vi "ImageProcessing_Main.vi"() -> ()   [LabVIEW 2020]
uses:
  #typedef_ImPro_InputData.ctl
  #typedef_states.ctl
  #typedef_ImagePath.ctl
panel:
  in  "Sharp":bool
  in  "Blur":bool
  in  "Gauss":bool
  in  "Binaryzacja":bool
  in  "stop":bool
  in  "Load Picture":bool
  in  "Path":path
  out "Output Image":picture
  out "Input Image":picture
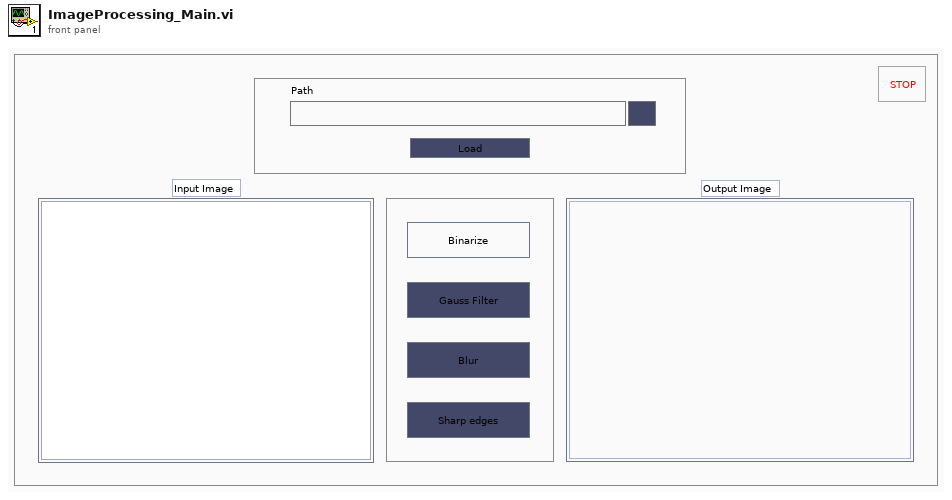
[diagram p1: front panel]
types:
  T1 = typedef "#typedef_ImagePath.ctl" = cluster{"Image path":path}
  T2 = typedef "#typedef_ImPro_InputData.ctl" = cluster{"Command":T3, "Data":variant}
  T3 = typedef "#typedef_states.ctl" = enum16{"Rozmycie", "Wyostrzenie", "Gauss", "Binaryzacja", "Load Picture", "Exit"}
  T4 = typedef "imagedata.ctl" = cluster{"image type":i32, "image depth":i32, "image":u8[], "mask":u8[], "colors":u32[], "Rectangle":cluster{"left":i16, "top":i16, "right":i16, "bottom":i16}}
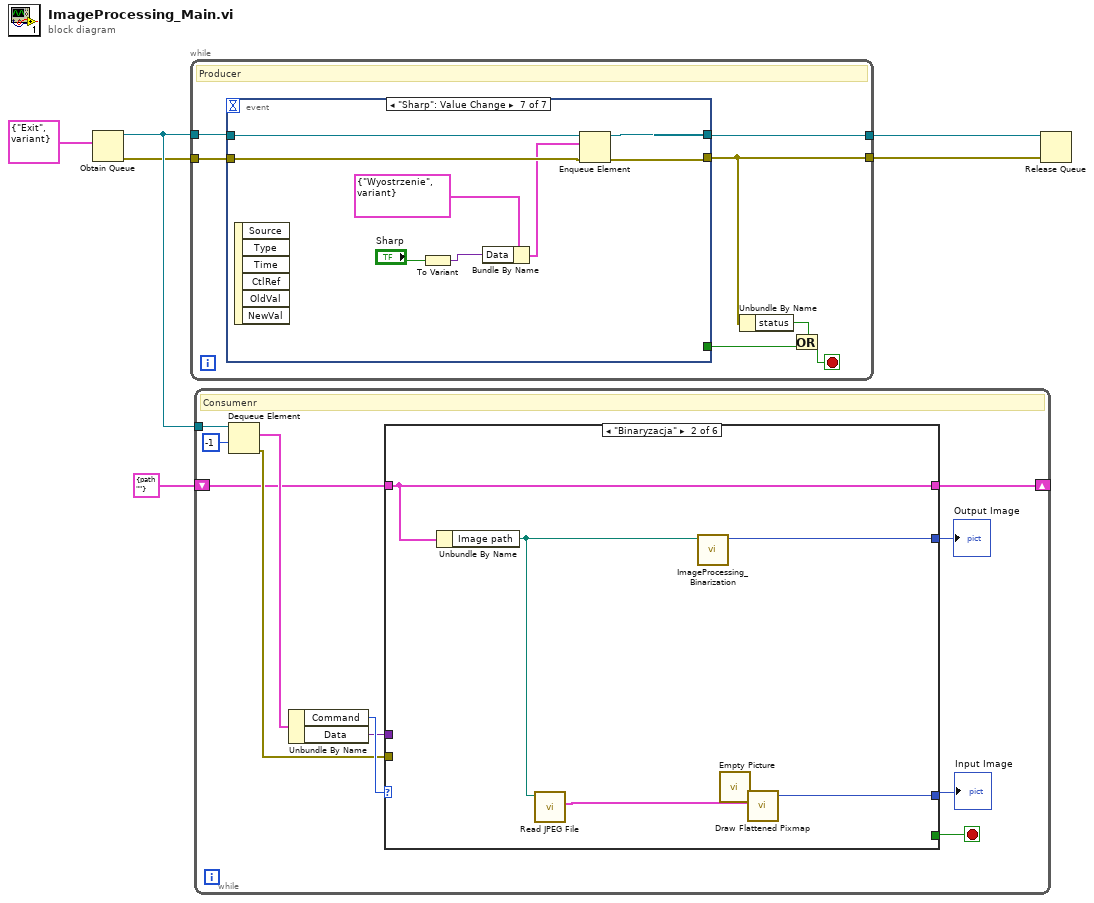
[diagram p0: block diagram]
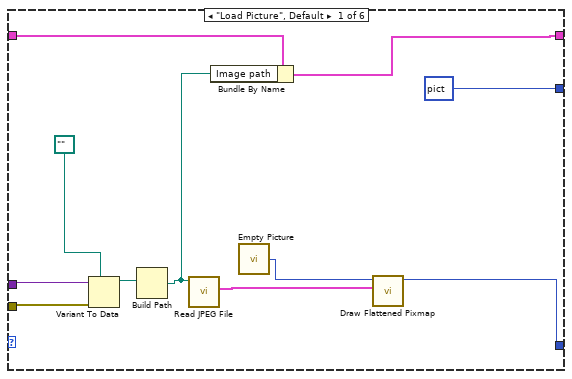
[diagram p2: hidden frame]
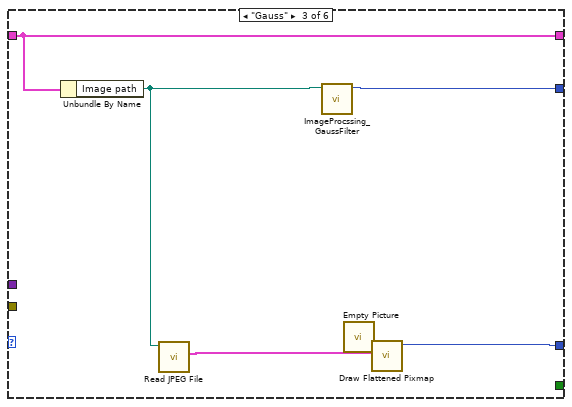
[diagram p3: hidden frame]
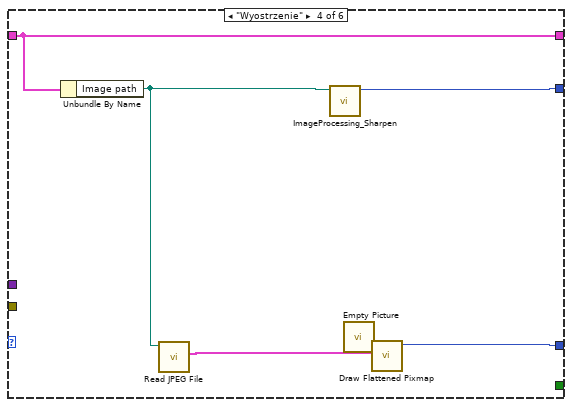
[diagram p4: hidden frame]
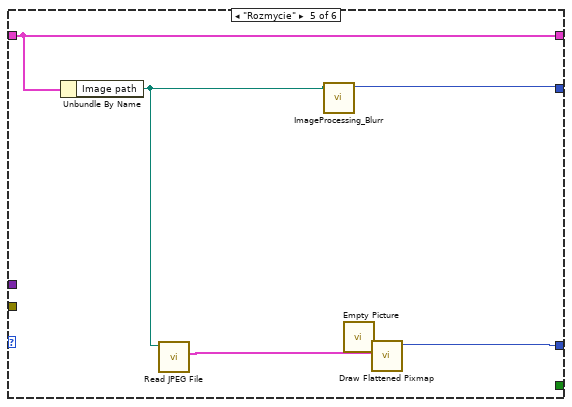
[diagram p5: hidden frame]
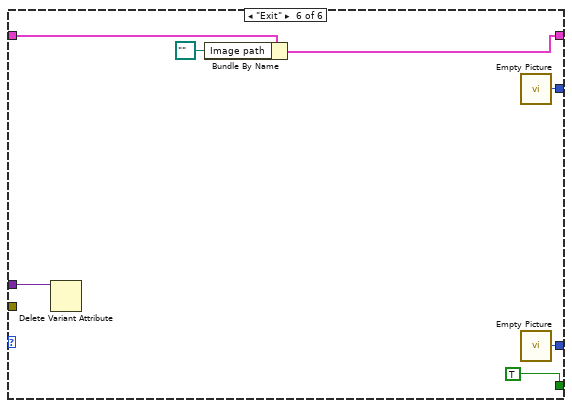
[diagram p6: hidden frame]
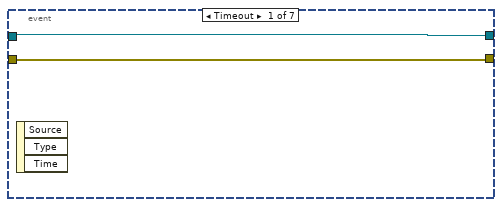
[diagram p7: hidden frame]
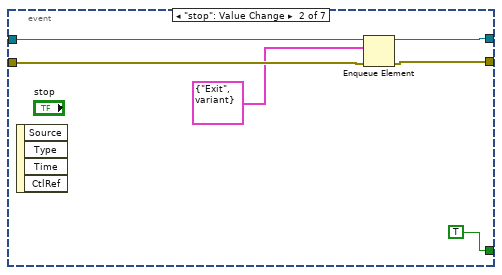
[diagram p8: hidden frame]
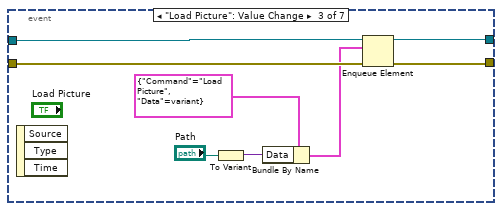
[diagram p9: hidden frame]
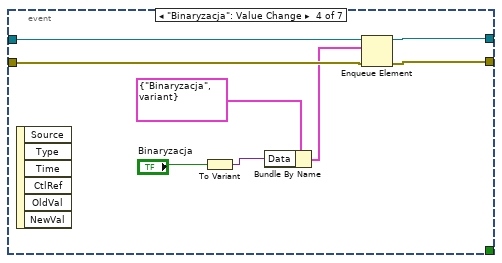
[diagram p10: hidden frame]
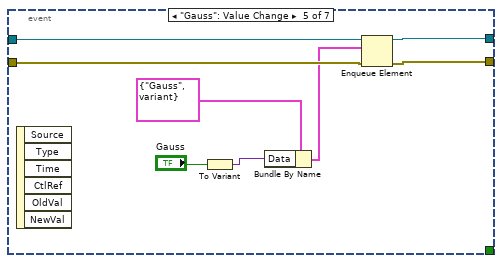
[diagram p11: hidden frame]
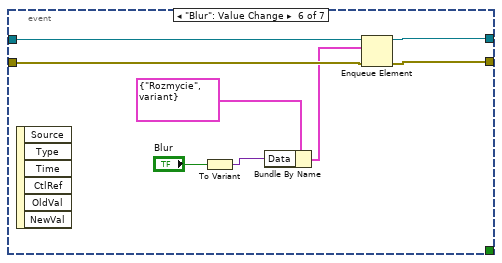
[diagram p12: hidden frame]
diagram:
  n1 = Obtain Queue(element data type=T2 {"Command"=enum."Exit", "Data"=variant} ("Input data")) -> (queue out=w5:refnum<queue>, error out=w4:errorcluster)  [unwired: 4 in, 1 out]
  n2 = while {
    tunnel: w5 -> [w13]
    tunnel: [w12] -> w6
    tunnel: w4 -> [w11]
    tunnel: [w8] -> w2
    stop <- w10 stop-if-true
    # "Producer"
    n3 = event shown="[6] \"Sharp\": Value Change" {
      selector: _ -> [_ _ _ _ _ _ _]
      dyn-events: _ -> [_ _ _ _ _ _ _]
      timeout: _ -> [_ _ _ _ _ _ _]
      tunnel: [w15 w21 w25 w34 w42 w50 w58] -> w12
      tunnel: w13 -> [w15 w18 w27 w36 w44 w52 w60]
      tunnel: w11 -> [w14 w20 w26 w35 w43 w51 w59]
      tunnel: [w14 w19 w24 w33 w41 w49 w57] -> w8
      tunnel: [_ TRUE ("stop") _ _ _ _ _] -> w9
      event Timeout {
        n4 = event-data() -> ()  [unwired: 1 in, 3 out]
      }
      event "stop": Value Change {
        n5 = event-data() -> ()  [unwired: 1 in, 4 out]
        n6 = Enqueue Element(queue=w18, element=T2 {"Command"=enum."Exit", "Data"=variant} ("Input data"), error in (no error)=w20) -> (queue out=w21:refnum<queue>, error out=w19:errorcluster)  [unwired: 1 in, 1 out]
      }
      event "Load Picture": Value Change {
        n7 = event-data() -> ()  [unwired: 1 in, 3 out]
        n8 = To Variant(anything="Path") -> (Variant=w22:variant)
        n9 = Bundle By Name(cluster=T2 {"Command"=enum."Load Picture", "Data"=variant} ("Input data"), "Data"=w22) -> (w23:T2)
        n10 = Enqueue Element(queue=w27, element=w23, error in (no error)=w26) -> (queue out=w25:refnum<queue>, error out=w24:errorcluster)  [unwired: 1 in, 1 out]
      }
      event "Binaryzacja": Value Change {
        n11 = event-data() -> ()  [unwired: 1 in, 6 out]
        n12 = To Variant(anything="Binaryzacja") -> (Variant=w31:variant)
        n13 = Bundle By Name(cluster=T2 {"Command"=enum."Binaryzacja", "Data"=variant} ("Input data"), "Data"=w31) -> (w30:T2)
        n14 = Enqueue Element(queue=w36, element=w30, error in (no error)=w35) -> (queue out=w34:refnum<queue>, error out=w33:errorcluster)  [unwired: 1 in, 1 out]
      }
      event "Gauss": Value Change {
        n15 = event-data() -> ()  [unwired: 1 in, 6 out]
        n16 = To Variant(anything="Gauss") -> (Variant=w40:variant)
        n17 = Bundle By Name(cluster=T2 {"Command"=enum."Gauss", "Data"=variant} ("Input data"), "Data"=w40) -> (w39:T2)
        n18 = Enqueue Element(queue=w44, element=w39, error in (no error)=w43) -> (queue out=w42:refnum<queue>, error out=w41:errorcluster)  [unwired: 1 in, 1 out]
      }
      event "Blur": Value Change {
        n19 = event-data() -> ()  [unwired: 1 in, 6 out]
        n20 = To Variant(anything="Blur") -> (Variant=w48:variant)
        n21 = Bundle By Name(cluster=T2 {"Command"=enum."Rozmycie", "Data"=variant} ("Input data"), "Data"=w48) -> (w47:T2)
        n22 = Enqueue Element(queue=w52, element=w47, error in (no error)=w51) -> (queue out=w50:refnum<queue>, error out=w49:errorcluster)  [unwired: 1 in, 1 out]
      }
      event "Sharp": Value Change {
        n23 = event-data() -> ()  [unwired: 1 in, 6 out]
        n24 = To Variant(anything="Sharp") -> (Variant=w56:variant)
        n25 = Bundle By Name(cluster=T2 {"Command"=enum."Wyostrzenie", "Data"=variant} ("Input data"), "Data"=w56) -> (w55:T2)
        n26 = Enqueue Element(queue=w60, element=w55, error in (no error)=w59) -> (queue out=w58:refnum<queue>, error out=w57:errorcluster)  [unwired: 1 in, 1 out]
      }
    }
    n27 = Unbundle By Name(w8) -> ("status"=w7:bool)
    n28 = Or(x=w7, y=w9) -> (x .or. y?=w10:bool)
  }
  n29 = while {
    tunnel: w5 -> [w72]
    shift-right: [w63] -> _
    shift-left: T1 {"Image path"=path ""} -> [w64]
    stop <- w66 stop-if-true
    # "Consumenr"
    n30 = Dequeue Element(queue=w72, timeout in ms (-1)=-1) -> (element=w71:T2, error out=w67:errorcluster)  [unwired: 1 in, 2 out]
    n31 = Unbundle By Name(w71) -> ("Command"=w70:T3, "Data"=w69:variant)
    n32 = case shown="\"Binaryzacja\"" w70 {
      tunnel: w69 -> [w83 _ _ _ _ w113]
      tunnel: w67 -> [w81 _ _ _ _ _]
      tunnel: [w78 w86 w92 w98 w104 w109] -> w65
      tunnel: [_ _ _ _ _ TRUE] -> w66
      tunnel: w64 -> [w76 w89 w95 w101 w107 w112]
      tunnel: [w75 w89 w95 w101 w107 w111] -> w63
      tunnel: [picture data[5B] ("new picture") w84 w90 w96 w102 w108] -> w62
      frame "Load Picture", Default {
        n33 = Variant To Data(error in=w81, type=path "", Variant=w83) -> (data=w80:path)  [unwired: 1 out]
        n34 = Build Path(name or relative path=w80) -> (appended path=w74:path)  [unwired: 1 in]
        n35 = call <vilib>:"Read JPEG File.vi"("path to JPEG file"=w74) -> ("image data"=w79:T4)  [unwired: 8 in, 2 out]
        n36 = Bundle By Name(cluster=w76, "Image path"=w74) -> (w75:T1)
        n37 = call "Empty Picture"() -> ("empty picture"=w77:picture)
        n38 = call <vilib>:"Draw Flattened Pixmap.vi"("image data"=w79, "picture"=w77) -> ("new picture"=w78:picture)  [unwired: 7 in]
      }
      frame "Binaryzacja" {
        n39 = Unbundle By Name(w89) -> ("Image path"=w85:path)
        n40 = call <vilib>:"Read JPEG File.vi"("path to JPEG file"=w85) -> ("image data"=w88:T4)  [unwired: 8 in, 2 out]
        n41 = call "ImageProcessing_Binarization.vi"("Path"=w85) -> ("Input Image"=w84:picture)  [unwired: 10 in]
        n42 = call "Empty Picture"() -> ("empty picture"=w87:picture)
        n43 = call <vilib>:"Draw Flattened Pixmap.vi"("image data"=w88, "picture"=w87) -> ("new picture"=w86:picture)  [unwired: 7 in]
      }
      frame "Gauss" {
        n44 = Unbundle By Name(w95) -> ("Image path"=w91:path)
        n45 = call <vilib>:"Read JPEG File.vi"("path to JPEG file"=w91) -> ("image data"=w94:T4)  [unwired: 8 in, 2 out]
        n46 = call "ImageProcssing_GaussFilter.vi"("Path"=w91) -> ("2D Picture"=w90:picture)  [unwired: 10 in]
        n47 = call "Empty Picture"() -> ("empty picture"=w93:picture)
        n48 = call <vilib>:"Draw Flattened Pixmap.vi"("image data"=w94, "picture"=w93) -> ("new picture"=w92:picture)  [unwired: 7 in]
      }
      frame "Wyostrzenie" {
        n49 = Unbundle By Name(w101) -> ("Image path"=w97:path)
        n50 = call <vilib>:"Read JPEG File.vi"("path to JPEG file"=w97) -> ("image data"=w100:T4)  [unwired: 8 in, 2 out]
        n51 = call "ImageProcessing_Sharpen.vi"("Path"=w97) -> ("2D Picture"=w96:picture)  [unwired: 10 in]
        n52 = call "Empty Picture"() -> ("empty picture"=w99:picture)
        n53 = call <vilib>:"Draw Flattened Pixmap.vi"("image data"=w100, "picture"=w99) -> ("new picture"=w98:picture)  [unwired: 7 in]
      }
      frame "Rozmycie" {
        n54 = Unbundle By Name(w107) -> ("Image path"=w103:path)
        n55 = call <vilib>:"Read JPEG File.vi"("path to JPEG file"=w103) -> ("image data"=w106:T4)  [unwired: 8 in, 2 out]
        n56 = call "ImageProcessing_Blurr.vi"("Path"=w103) -> ("2D Picture"=w102:picture)  [unwired: 10 in]
        n57 = call "Empty Picture"() -> ("empty picture"=w105:picture)
        n58 = call <vilib>:"Draw Flattened Pixmap.vi"("image data"=w106, "picture"=w105) -> ("new picture"=w104:picture)  [unwired: 7 in]
      }
      frame "Exit" {
        n59 = Delete Variant Attribute(7:w113) -> ()  [unwired: 2 in, 3 out]
        n60 = Bundle By Name(cluster=w112, "Image path"=path "") -> (w111:T1)
        n61 = call "Empty Picture"() -> ("empty picture"=w108:picture)
        n62 = call "Empty Picture"() -> ("empty picture"=w109:picture)
      }
    }
    "Input Image" <- w65
    "Output Image" <- w62
  }
  n63 = Release Queue(queue=w6, error in (no error)=w2) -> ()  [unwired: 1 in, 3 out]
